vi "Read Line.vi"() -> ()   [LabVIEW 2013]
uses:
  <vilib>/NXT/Block Support/NXT_InputPort.ctl
  <vilib>/NXT/Dual Mode Library/Display/drawNumber.vi
  <vilib>/NXT/Dual Mode Library/Sound/Tone.vi
panel:
  out "Blue Line":i16
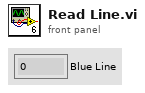
[diagram p1: front panel]
types:
  T1 = typedef "NXT_InputPort.ctl" = u32
  T2 = typedef "LVHSConnector.ctl" = refnum<class "BrickReference.lvclass">
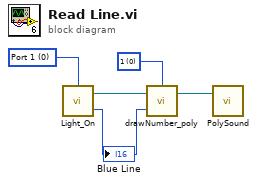
[diagram p0: block diagram]
diagram:
  w3 = i16 0 items=["1", "2", "3", "4", "5", "6", "7", "8", "9", "10", "11", "12"] ("Line")
  w5 = T1 0 items=["Port 1", "Port 2", "Port 3", "Port 4"] ("Port (Port 3)")
  n1 = call <vilib>:"Light_On.vi"("Port (Port 3)"=w5) -> ("Scaled Value"=w4:i16, "NXT/EV3"=w2:T2)  [unwired: 2 in]
  "Blue Line" <- w4
  n2 = call-poly <vilib>:"drawNumber_poly.vi"("number"=w4, "NXT/EV3"=w2, "Line"=w3) -> ("NXT/EV3"=w1:T2)  [unwired: 1 in]
  n3 = call-poly <vilib>:"PolySound.vi"("NXT/EV3"=w1) -> ()  [unwired: 3 in, 1 out]
